vi "edit_coating_1.vi"() -> ()   [LabVIEW 2009]
panel:
  in  "Edit":bool caption="OK2"
  in  "Delete":bool caption="OK2"
  in  "Cancel":bool
  in  "Recipe List":i32(listbox)
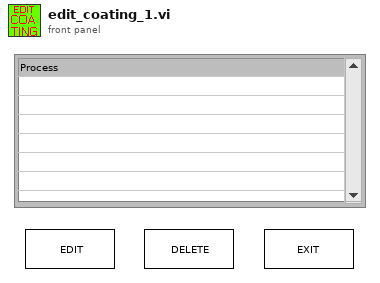
[diagram p1: front panel]
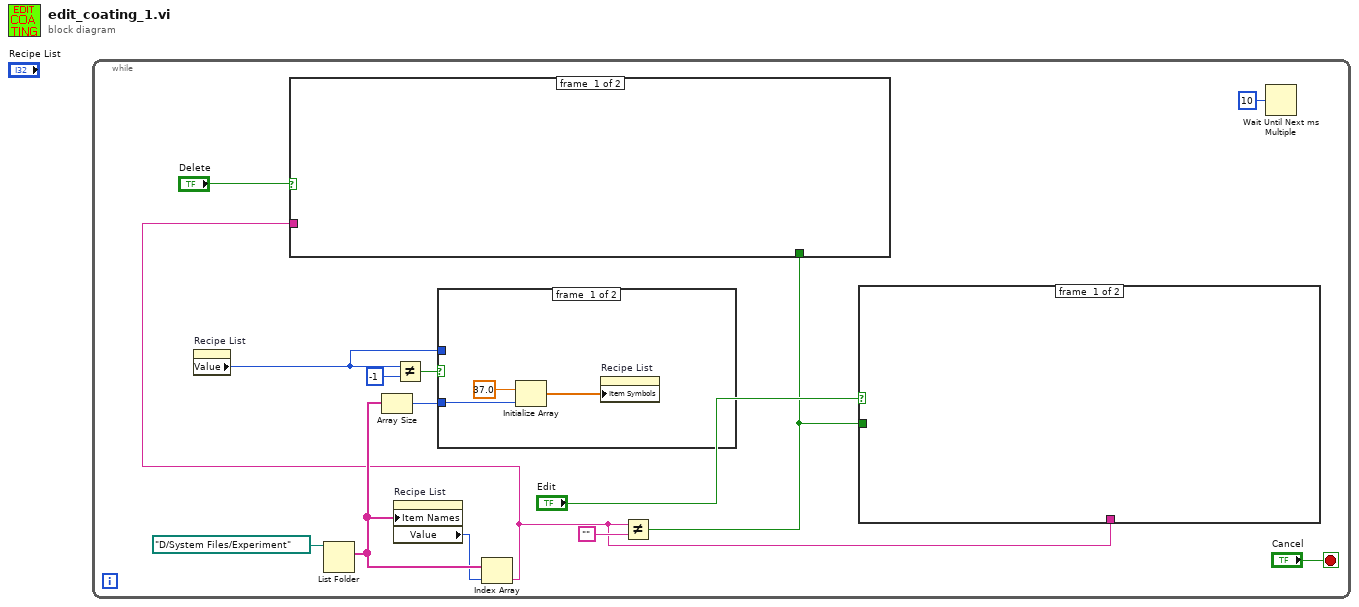
[diagram p0: block diagram]
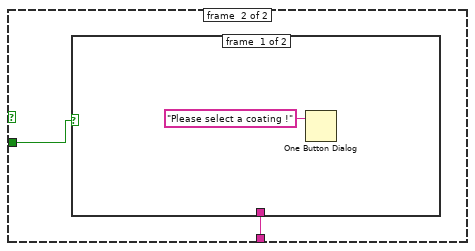
[diagram p2: hidden frame]
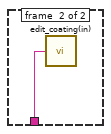
[diagram p3: hidden frame]
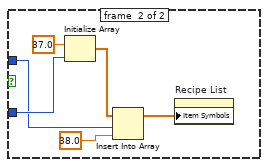
[diagram p4: hidden frame]
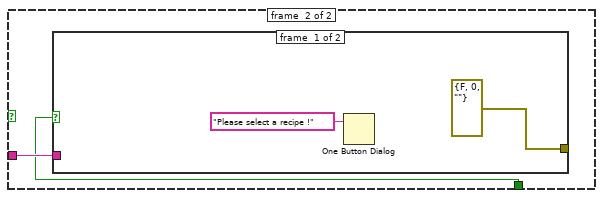
[diagram p5: hidden frame]
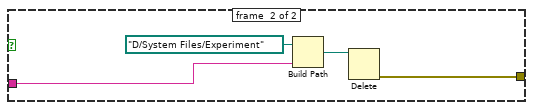
[diagram p6: hidden frame]
diagram:
  n1 = while {
    stop <- "Cancel" stop-if-true
    n2 = property on="Recipe List" class="LstBox (strict)"() -> ("Value"=w9:i32)  [unwired: 2 in, 2 out]
    n3 = List Folder(path=path "D:/System Files/Experiment") -> (filenames=w8:string[])  [unwired: 3 in, 3 out]
    n4 = Array Size(array=w8) -> (size(s)=w10:i32)
    n5 = property on="Recipe List" class="LstBox (strict)"("Item Names"=w8) -> ("Value"=w7:i32)  [unwired: 2 in, 2 out]
    n6 = Not Equal?(x=w9, y=-1) -> (x != y?=w11:bool)
    n7 = case shown="False" w11 {
      tunnel: w10 -> [w20 w25]
      tunnel: w9 -> [_ w24]
      frame #0 {
        n8 = Initialize Array(37.0 ("element"), w20) -> (w19:dbl[])
        n9 = property on="Recipe List" class="LstBox (strict)"("Item Symbols"=w19) -> ()  [unwired: 2 in, 2 out]
      }
      frame #1 {
        n10 = Initialize Array(37.0 ("element"), w25) -> (w27:dbl[])
        n11 = Insert Into Array(array=w27, index=w24, new element=38.0 ("element")) -> (w22:dbl[])
        n12 = property on="Recipe List" class="LstBox (strict)"("Item Symbols"=w22) -> ()  [unwired: 2 in, 2 out]
      }
    }
    n13 = Index Array(array=w8, index=w7) -> (element=w4:string)
    n14 = Not Equal?(x=w4, y="") -> (x != y?=w3:bool)
    n15 = case shown="True" "Delete" {
      tunnel: w4 -> [_ w29]
      tunnel: w3 -> [_ w28]
      frame #0 {
      }
      frame #1 {
        n16 = case shown="True" w28 {
          tunnel: w29 -> [_ w35]
          tunnel: [errorcluster {"status"=FALSE, "code"=0, "source"=""} ("error out") w32] -> _
          frame #0 {
            n17 = One Button Dialog(message="Please select a recipe !") -> ()  [unwired: 1 in, 1 out]
          }
          frame #1 {
            n18 = Build Path(base path=path "D:/System Files/Experiment", name or relative path=w35) -> (appended path=w34:path)
            n19 = Delete(path (use dialog)=w34) -> (error out=w32:errorcluster)  [unwired: 4 in, 2 out]
          }
        }
      }
    }
    n20 = case shown="True" "Edit" {
      tunnel: w4 -> [_ w16]
      tunnel: w3 -> [_ w15]
      frame #0 {
      }
      frame #1 {
        n21 = case shown="True" w15 {
          tunnel: w16 -> [_ w18]
          frame #0 {
            n22 = One Button Dialog(message="Please select a coating !") -> ()  [unwired: 1 in, 1 out]
          }
          frame #1 {
            n23 = call "edit_coating(in).vi"("Path"=w18) -> ()
          }
        }
      }
    }
    n24 = Wait Until Next ms Multiple(millisecond multiple=u32 10) -> ()  [unwired: 1 out]
  }
